vi "format_layer.vi"(2 "Repeats":i32, 3 "Input cluster":T3 {"T (Å) / D (s)" format="%.1f"; "Elements" items=["none"=0, "Se"=2, "Ti"=3, "Sn"=4]}, 4 "Source":T1) -> (0 "Output cluster":T2, 1 "Listbox text":string[](array[string]))   [LabVIEW 2012]
uses:
  <vilib>/Utility/miscctls.llb/LVStringsAndValuesArrayTypeDef_U16.ctl
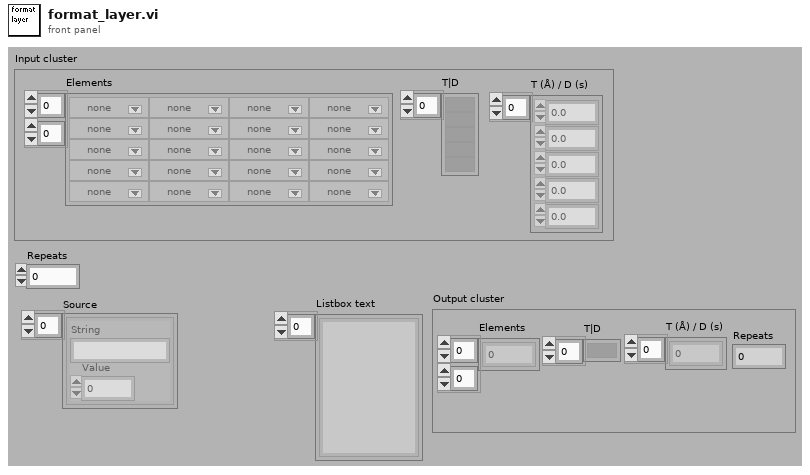
[diagram p1: front panel]
types:
  T1 = typedef "LVStringsAndValuesArrayTypeDef_U16.ctl" = cluster{"String":string, "Value":u16}[]
  T2 = cluster{"Elements":u16[][], "T|D":bool[], "T (Å) / D (s)":sgl[], "Repeats":i32}
  T3 = cluster{"Elements":u16[][], "T|D":bool[], "T (Å) / D (s)":sgl[]}
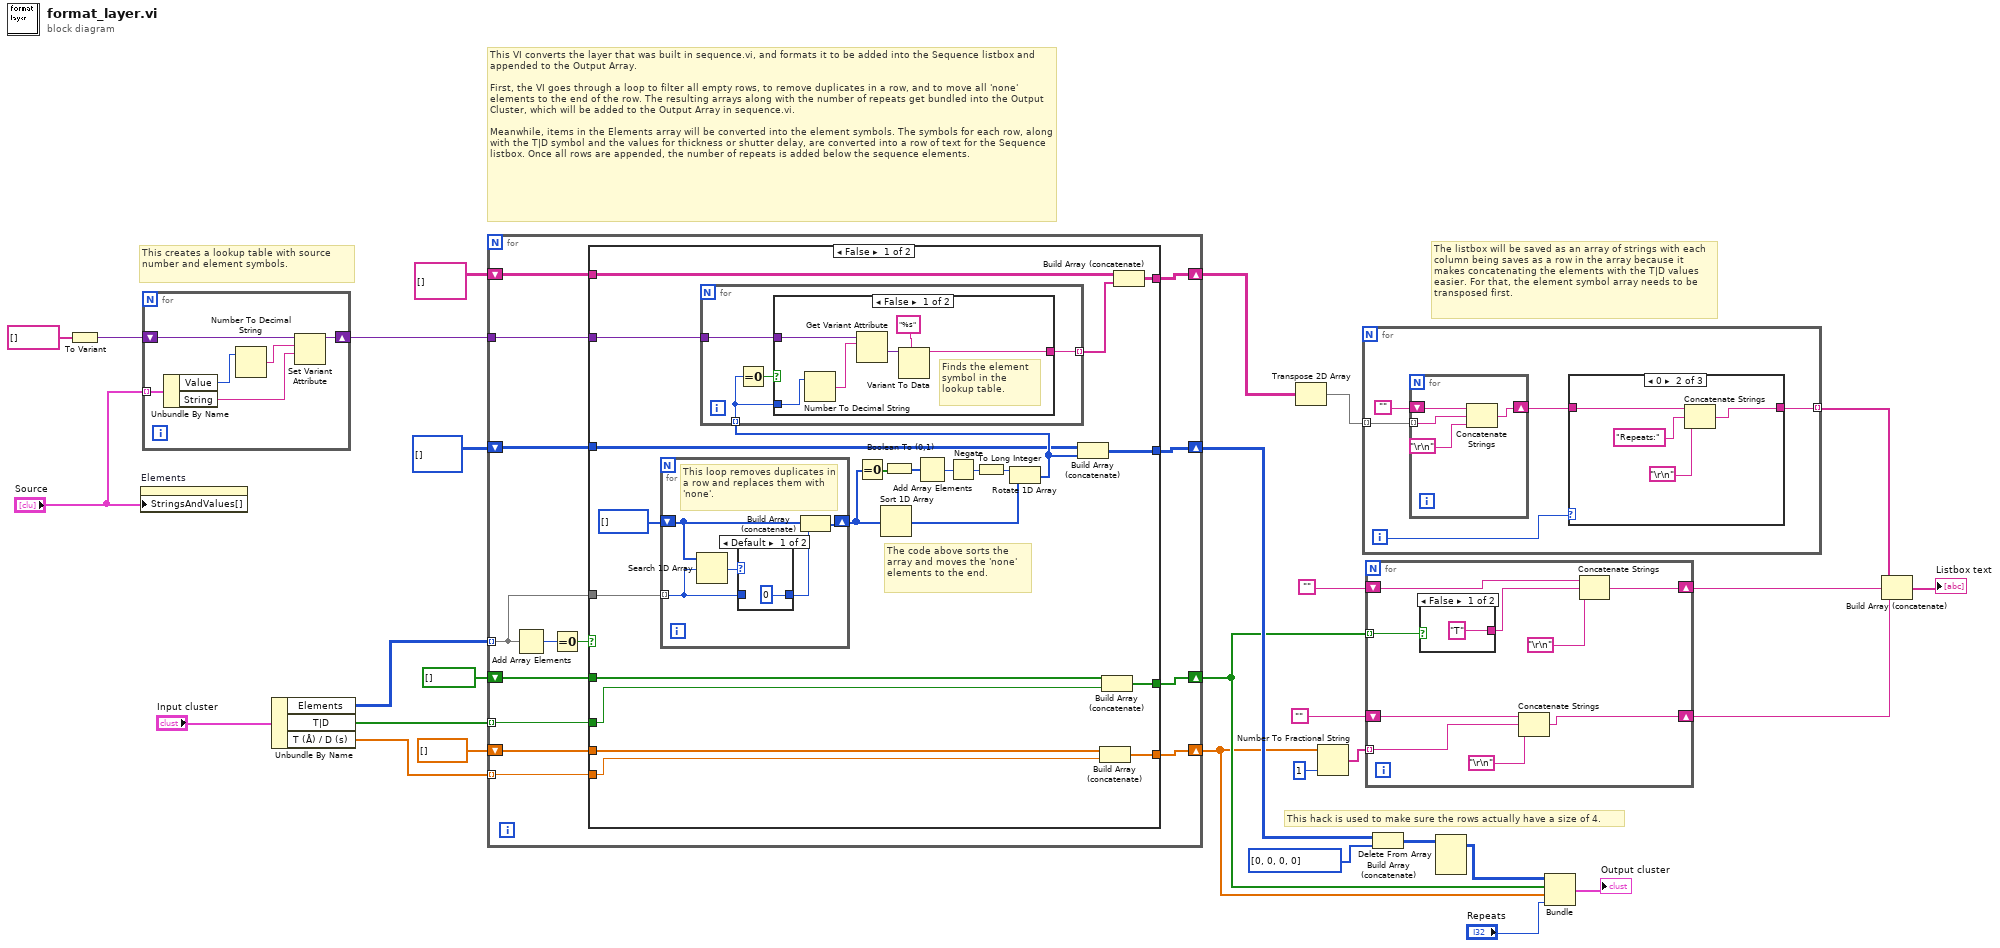
[diagram p0: block diagram]
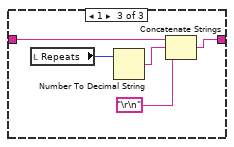
[diagram p3: hidden frame]
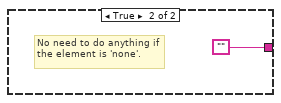
[diagram p4: hidden frame]
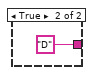
[diagram p7: hidden frame]
diagram:
  # "This hack is used to make sure the rows actually have a size of 4."
  # "The listbox will be saved as an array of strings with each column being saves as a row in the array because it makes concatenating the elements with the T|D values easier. For that, the element symbol array needs to be transposed first."
  # "This creates a lookup table with source number and element symbols."
  # "This VI converts the layer that was built in sequence.vi, and formats it to be added into the Sequence listbox and appended to the Output Array.\n\nFirst, the VI goes through a loop to filter all empty rows, to remove duplicates in a row, and to move all 'none' elements to the end of the row. The resulting arrays along with the number of repeats get bundled into the Output Cluster, which will be added to the Output Array in sequence.vi.\n\nMeanwhile, items in the Elements array will be converted into the element symbols. The symbols for each row, along with the T|D symbol and the values for thickness or shutter delay, are converted into a row of text for the Sequence listbox. Once all rows are appended, the number of repeats is added below the sequence elements."
  n1 = To Variant(anything=string[] []) -> (Variant=w13:variant)
  n2 = property on="Elements" class="Ring (strict)"("StringsAndValues[]"="Source") -> ()  [unwired: 2 in, 2 out]
  n3 = for {
    tunnel: "Source" -> [w36] mode=indexing
    shift-right: [w31] -> w14
    shift-left: w13 -> [w32]
    n4 = Unbundle By Name(w36) -> ("Value"=w35:u16, "String"=w33:string)
    n5 = Number To Decimal String(number=w35) -> (decimal integer string=w34:string)  [unwired: 1 in]
    n6 = Set Variant Attribute(Variant=w32, name=w34, value=w33) -> (Variant out=w31:variant)  [unwired: 1 in, 2 out]
  }
  n7 = Unbundle By Name("Input cluster") -> ("Elements"=w29:u16[][], "T|D"=w23:bool[], "T (Å) / D (s)"=w22:sgl[])
  n8 = for {
    tunnel: w29 -> [w48] mode=indexing
    tunnel: w23 -> [w47] mode=indexing
    tunnel: w22 -> [w46] mode=indexing
    tunnel: w14 -> [w45]
    shift-right: [w43] -> w9
    shift-left: bool[] [] -> [w40]
    shift-right: [w42] -> w8
    shift-left: dbl[] [] -> [w41]
    shift-right: [w44] -> w10
    shift-left: u16[][] [] -> [w39]
    shift-right: [w37] -> w11
    shift-left: string[][] [] -> [w38]
    n9 = Add Array Elements(numeric array=w48) -> (sum=w50:u16)
    n10 = Equal To 0?(x=w50) -> (x = 0?=w49:bool)
    n11 = case shown="False" w49 {
      tunnel: w48 -> [w72 _]
      tunnel: [w58 w92] -> w43
      tunnel: [w63 w91] -> w42
      tunnel: w47 -> [w60 _]
      tunnel: w46 -> [w61 _]
      tunnel: [w57 w94] -> w44
      tunnel: w45 -> [w64 _]
      tunnel: w41 -> [w62 w91]
      tunnel: w40 -> [w59 w92]
      tunnel: w39 -> [w55 w94]
      tunnel: w38 -> [w54 w93]
      tunnel: [w53 w93] -> w37
      frame False {
        # "The code above sorts the array and moves the 'none' elements to the end."
        n12 = for {
          tunnel: w72 -> [w87] mode=indexing
          shift-right: [w86] -> w65
          shift-left: u16[] [] -> [w85]
          # "This loop removes duplicates in a row and replaces them with 'none'."
          n13 = Search 1D Array(1D array=w85, element=w87) -> (index of element=w88:i32)  [unwired: 1 in]
          n14 = case shown="Default" w88 {
            tunnel: w87 -> [_ w90]
            tunnel: [u16 0 w90] -> w84
            frame Default {
            }
            frame -1 {
            }
          }
          n15 = Build Array (concatenate)(w85, w84) -> (w86:u16[])
        }
        n16 = Equal To 0?(x=w65) -> (x = 0?=w66:bool[])
        n17 = Sort 1D Array(array=w65) -> (sorted array=w70:u16[])
        n18 = Boolean To (0,1)(Boolean=w66) -> (0, 1=w67:i16[])
        n19 = Add Array Elements(numeric array=w67) -> (sum=w68:i16)
        n20 = Negate(x=w68) -> (-x=w69:i16)
        n21 = To Long Integer(number=w69) -> (32bit integer=w51:i32)
        n22 = Rotate 1D Array(1:w70, 2:w51) -> (0:w56:u16[])
        n23 = for {
          tunnel: w56 -> [w75] mode=indexing
          tunnel: w64 -> [w74]
          tunnel: [w73] -> w52 mode=indexing
          n24 = Equal To 0?(x=w75) -> (x = 0?=w76:bool)
          n25 = case shown="False" w76 {
            tunnel: [w79 ""] -> w73
            tunnel: w75 -> [w78 _]
            tunnel: w74 -> [w82 _]
            frame False {
              # "Finds the element symbol in the lookup table."
              n26 = Number To Decimal String(number=w78) -> (decimal integer string=w77:string)  [unwired: 1 in]
              n27 = Get Variant Attribute(Variant=w82, name=w77) -> (value=w81:variant)  [unwired: 2 in, 3 out]
              n28 = Variant To Data(type="%s", Variant=w81) -> (data=w79:string)  [unwired: 1 in, 1 out]
            }
            frame True {
              # "No need to do anything if the element is 'none'."
            }
          }
        }
        n29 = Build Array (concatenate)(w55, w56) -> (w57:u16[][])
        n30 = Build Array (concatenate)(w62, w61) -> (w63:dbl[])
        n31 = Build Array (concatenate)(w59, w60) -> (w58:bool[])
        n32 = Build Array (concatenate)(w54, w52) -> (w53:string[][])
      }
      frame True {
        # "If the sum of all elements in a row is zero, then all elements are 'none', so do nothing and don't append the T|D values."
      }
    }
  }
  n33 = Transpose 2D Array(2D array=w11) -> (transposed array=w24:string[][])
  n34 = Number To Fractional String(number=w8, precision (6)=1) -> (F-format string=w28:string[])  [unwired: 2 in]
  n35 = for {
    tunnel: w24 -> [w98] mode=indexing
    tunnel: [w95] -> w7 mode=indexing
    i -> [w96]
    n36 = for {
      shift-right: [w112] -> w97
      shift-left: "" -> [w111]
      tunnel: w98 -> [w110] mode=indexing
      n37 = Concatenate Strings(w111, w110, "\r\n") -> (w112:string)
    }
    n38 = case shown="0" w96 {
      tunnel: w97 -> [w100 w103 w108]
      tunnel: [w100 w104 w107] -> w95
      frame 2, Default {
      }
      frame 0 {
        n39 = Concatenate Strings(w103, "Repeats:", "\r\n") -> (w104:string)
      }
      frame 1 {
        n40 = local read "Repeats"() -> (w105:i32)
        n41 = Number To Decimal String(number=w105) -> (decimal integer string=w106:string)  [unwired: 1 in]
        n42 = Concatenate Strings(w108, w106, "\r\n") -> (w107:string)
      }
    }
  }
  n43 = for {
    shift-right: [w121] -> w15
    shift-left: "" -> [w122]
    tunnel: w28 -> [w118] mode=indexing
    shift-right: [w116] -> w25
    shift-left: "" -> [w117]
    tunnel: w9 -> [w114] mode=indexing
    n44 = case shown="False" w114 {
      tunnel: ["T" "D"] -> w120
      frame False {
      }
      frame True {
      }
    }
    n45 = Concatenate Strings(w117, w118, "\r\n") -> (w116:string)
    n46 = Concatenate Strings(w122, w120, "\r\n") -> (w121:string)
  }
  n47 = Build Array (concatenate)(w10, u16[] [0, 0, 0, 0]) -> (w17:u16[][])
  n48 = Delete From Array(array=w17) -> (array with subset deleted=w16:u16[][])  [unwired: 3 in, 1 out]
  n49 = Bundle(w16, w9, w8, "Repeats"="Repeats") -> (→"Output cluster":cluster{u16[][], bool[], dbl[], "Repeats":i32})  [unwired: 1 in]
  n50 = Build Array (concatenate)(w7, w15, w25) -> (→"Listbox text":string[])
